vi "Create File Stream Content.vi"(5 "HttpContent_Stream in":refnum<class "HttpContent_Stream.lvclass">, 8 "error in (no error)":errorcluster, 11 "File":path) -> (0 "error out":errorcluster, 3 "HttpContent_Stream out":refnum<class "HttpContent_Stream.lvclass">)   [LabVIEW 2018, in "HttpClient_NET.lvlib" / "HttpContent_Stream.lvclass"]
uses:
  HttpContent_Stream.lvclass
  Types/HttpNet_error_enum.ctl
  HttpClient_NET.lvlib
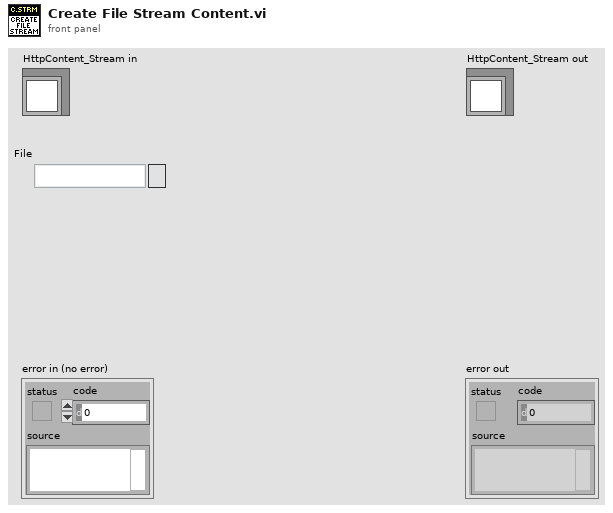
[diagram p1: front panel]
types:
  T1 = typedef "HttpClient_NET.lvlib/HttpNet_error_enum.ctl" = enum16{"REST method is not available", "URL cannot be blank", "Output filepath cannot be empty", "Input filepath cannot be empty", "Internal .NET error %s", "Output filepath cannot be directory", "Download Task no longer exists", "Mutipart Put not supported from REST Client Interface.  Please revert to lower level classes"}
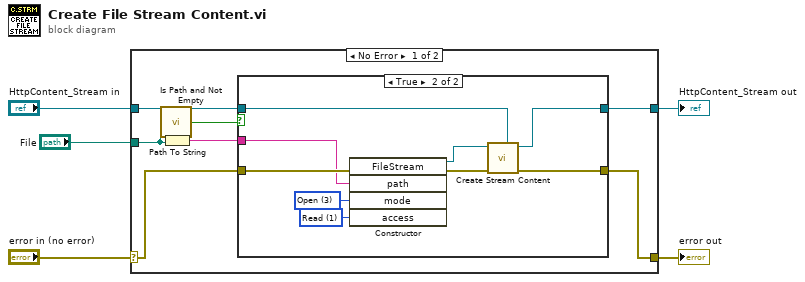
[diagram p0: block diagram]
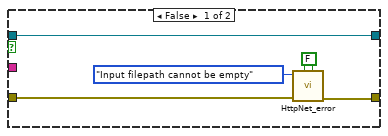
[diagram p2: hidden frame]
diagram:
  n1 = case shown="No Error" "error in (no error)" {
    selector: "error in (no error)" -> [w10 w28]
    tunnel: [w9 w28] -> w4
    tunnel: [w11 w27] -> w2
    tunnel: "HttpContent_Stream in" -> [w12 w27]
    tunnel: "File" -> [w7 _]
    frame No Error {
      n2 = call <vilib>:"Is Path and Not Empty.vi"("path"=w7) -> ("Is Path and Not Empty?"=w6:bool)  [unwired: 4 in]
      n3 = Path To String(path=w7) -> (string=w8:string)
      n4 = case shown="True" w6 {
        tunnel: w12 -> [w17 w22]
        tunnel: [w17 w21] -> w11
        tunnel: w10 -> [w14 w20]
        tunnel: [w13 w19] -> w9
        tunnel: w8 -> [_ w18]
        frame False {
          w15 = FALSE ("OverrideExistingErrors [T]")
          n5 = call "HttpNet_error.vi"("ShowCallChain [T]"=w15, "OverrideExistingErrors [T]"=w15, "Error In"=w14, "Error"=HttpNet_error_enum."Input filepath cannot be empty") -> ("Error Out"=w13:errorcluster)  [unwired: 7 in]
        }
        frame True {
          w25 = 1 items=["Read"=1, "Write"=2, "ReadWrite"=3] ("access")
          w26 = 3 items=["CreateNew"=1, "Create"=2, "Open"=3, "OpenOrCreate"=4, "Truncate"=5, "Append"=6] ("mode")
          n6 = constructor class="FileStream"(error in=w20, "path"=w18, "mode"=w26, "access"=w25) -> (reference out=w23:refnum<k24>, error out=w24:errorcluster)  [unwired: 2 in, 4 out]
          n7 = call "Create Stream Content.vi"("HttpContent_Stream in"=w22, "error in (no error)"=w24, "content"=w23) -> ("error out"=w19:errorcluster, "HttpContent_Stream out"=w21:refnum<class "HttpContent_Stream.lvclass">)  [unwired: 7 in]
        }
      }
    }
    frame Error {
    }
  }
  "error out" <- w4
  "HttpContent_Stream out" <- w2
